vi "SaveLoadGameBoard.vi"(8 "error in (no error)":errorcluster, 10 "mode":enum16{"Save", "Load"}(ring), 11 "Board in":T1[][](array[typedef])) -> (0 "error out":errorcluster, 2 "new file path (Not A Path if cancelled)":path, 3 "Board out":T1[][](array[typedef]))   [LabVIEW 2020]
doc: "This VI saves an array as CSV file via a dialog box or loads one from a file depending on save/load option. \nIt will return not a path constant if dialog is canceled but it won't throw an error."
uses:
  TypeDef/tiles-key.ctl
  <vilib>/Utility/file.llb/Write Delimited Spreadsheet (I64).vi
  <vilib>/Utility/file.llb/Read Delimited Spreadsheet (I64).vi
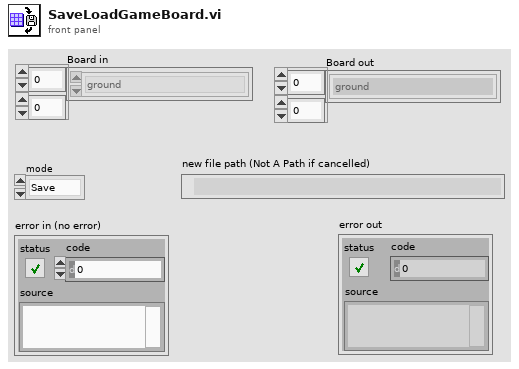
[diagram p1: front panel]
types:
  T1 = typedef "tiles-key.ctl" = enum16{"ground", "wall", "head (right)", "head (up)", "head (left)", "head (down)", "L-turn (right-up)", "L-turn (up-left)", "L-turn (left-down)", "L-turn (down-right)", "body (right)", "body (up)", "body (left)", "body (down)", "R-turn (right-down)", "R-turn (up-right)", "R-turn (left-up)", "R-turn (down-left)", "tail (right)", "tail (up)", "tail (left)", "tail (down)", "dead head (right)", "dead head (up)", "dead head (left)", "dead head (down)", "dead L-turn (right-up)", "dead L-turn (up-left)", "dead L-turn (left-down)", "dead L-turn (down-right)", "dead body (right)", "dead body (up)", "dead body (left)", "dead body (down)", "dead R-turn (right-down)", "dead R-turn (up-right)", "dead R-turn (left-up)", "dead R-turn (down-left)", "dead tail (right)", "dead tail (up)", "dead tail (left)", "dead tail (down)", "target red", "target blue", "target yellow", "target green"}
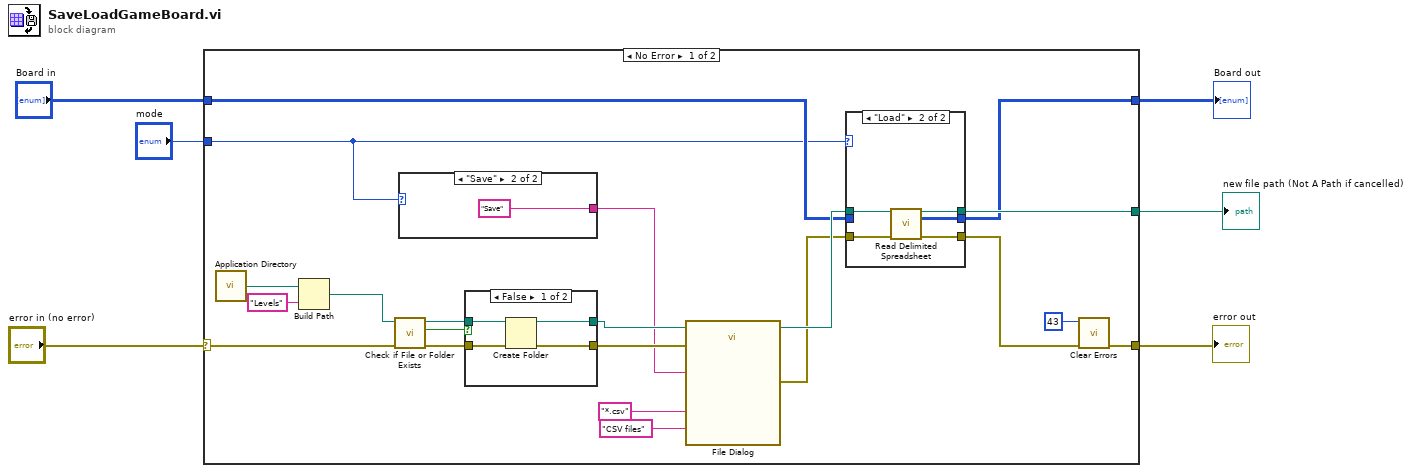
[diagram p0: block diagram]
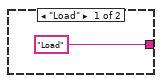
[diagram p2: hidden frame]
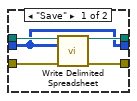
[diagram p4: hidden frame]
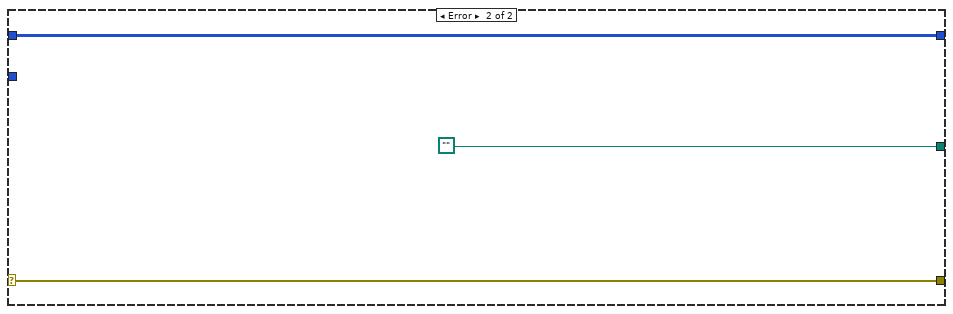
[diagram p5: hidden frame]
diagram:
  n1 = case shown="No Error" "error in (no error)" {
    selector: "error in (no error)" -> [w15 w47]
    tunnel: "Board in" -> [w26 w48]
    tunnel: [w24 path ""] -> w5
    tunnel: [w22 w47] -> w4
    tunnel: [w16 w48] -> w2
    tunnel: "mode" -> [w8 _]
    frame No Error {
      n2 = call <vilib>:"Application Directory.vi"() -> ("Application Directory"=w20:path)
      n3 = Build Path(base path=w20, name or relative path="Levels" ("string")) -> (appended path=w14:path)
      n4 = call <vilib>:"Check if File or Folder Exists.vi"("error in (no error)"=w15, "path"=w14) -> ("error out"=w9:errorcluster, "file or folder exists?"=w13:bool, "dup path"=w12:path)  [unwired: 7 in]
      n5 = case shown="\"Save\"" w8 {
        tunnel: ["Load" "Save"] -> w7
        frame "Load" {
        }
        frame "Save" {
        }
      }
      n6 = case shown="False" w13 {
        tunnel: w12 -> [w33 w35]
        tunnel: [w31 w35] -> w11
        tunnel: [w30 w34] -> w10
        tunnel: w9 -> [w32 w34]
        frame False {
          n7 = Create Folder(path (use dialog)=w33, error in=w32) -> (created path=w31:path, error out=w30:errorcluster)  [unwired: 1 in, 1 out]
        }
        frame True {
        }
      }
      n8 = call "File Dialog"("start path"=w11, "button label"=w7, "error in"=w10, "pattern (all files)"="*.csv", "pattern label"="CSV files") -> ("selected path"=w27:path, "error out"=w25:errorcluster)  [unwired: 7 in, 2 out]
      n9 = case shown="\"Load\"" w8 {
        tunnel: w27 -> [w40 w45]
        tunnel: w26 -> [w36 _]
        tunnel: w25 -> [w39 w44]
        tunnel: [w38 w42] -> w24
        tunnel: [w37 w43] -> w23
        tunnel: [w36 w41] -> w16
        frame "Save" {
          n10 = call-poly <vilib>:"Write Delimited Spreadsheet.vi"("file path (dialog if empty)"=w40, "2D data"=w36, "error in (no error)"=w39) -> ("new file path (Not A Path if cancelled)"=w38:path, "error out"=w37:errorcluster)  [unwired: 11 in]
        }
        frame "Load" {
          n11 = call-poly <vilib>:"Read Delimited Spreadsheet.vi"("file path (dialog if empty)"=w45, "error in (no error)"=w44) -> ("new file path (Not A Path if cancelled)"=w42:path, "all rows"=w41:i64[][], "error out"=w43:errorcluster)  [unwired: 8 in, 3 out]
        }
      }
      n12 = call <vilib>:"Clear Errors.vi"("error in (no error)"=w23, "specific error code to clear (0: all)"=43) -> ("error out"=w22:errorcluster)  [unwired: 4 in, 1 out]
    }
    frame Error {
    }
  }
  "error out" <- w4
  "new file path (Not A Path if cancelled)" <- w5
  "Board out" <- w2
